vi "Write Debug Mode.vi"(8 "error in (no error)":errorcluster, 10 "Debug Mode?":bool, 11 "Logger in":refnum<class "Logger.lvclass">) -> (0 "error out":errorcluster, 3 "Logger out":refnum<class "Logger.lvclass">)   [LabVIEW 2016, in "Logger.lvclass"]
uses:
  Logger.lvclass
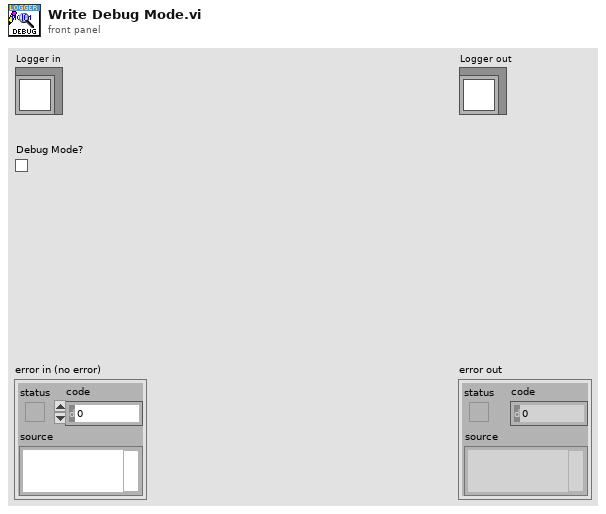
[diagram p1: front panel]
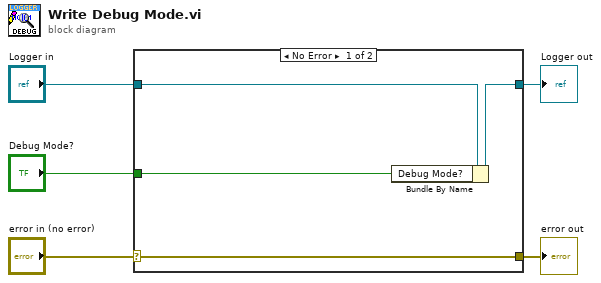
[diagram p0: block diagram]
diagram:
  n1 = case shown="No Error" "error in (no error)" {
    selector: "error in (no error)" -> [w9 w10]
    tunnel: [w9 w10] -> w4
    tunnel: [w6 w11] -> w2
    tunnel: "Logger in" -> [w8 w11]
    tunnel: "Debug Mode?" -> [w7 _]
    frame No Error {
      n2 = Bundle By Name(cluster=w8, "Debug Mode?"=w7) -> (w6:refnum<class "Logger.lvclass">)
    }
    frame Error {
    }
  }
  "error out" <- w4
  "Logger out" <- w2
